vi "Refresh DiffIO Listbox.vi"(8 "Filters":sgl[](array[numeric]), 9 "Names":string[](array[string]), 10 "Setup":T1[](array[typedef]) caption="Differential I/O Setup" {"Skip Fire Index" max=7; "Angles"."Duration [s]" format="%#_3p"; "Frequency [Hz]" format="%#_3p"}, 11 "MulticolumnListbox in":refnum<vi>) -> ()   [LabVIEW 2016, in "DCM System Explorer.lvlib"]
uses:
  DCM System Explorer.lvlib
  <vilib>/Powertrain Controls/Device Drivers/DCM/Diff IO/RT/Setup.ctl
  <vilib>/Powertrain Controls/Device Drivers/DCM/Diff IO/FPGA/Mode.ctl
  <vilib>/Powertrain Controls/Device Drivers/DCM/Diff IO/RT/Angle Control.ctl
  <vilib>/Powertrain Controls/Device Drivers/DCM/Diff IO/RT/DCM - RT - Diff IO.lvlib
  <vilib>/Powertrain Controls/Device Drivers/DCM/Diff IO/FPGA/DCM - FPGA - Diff IO.lvlib
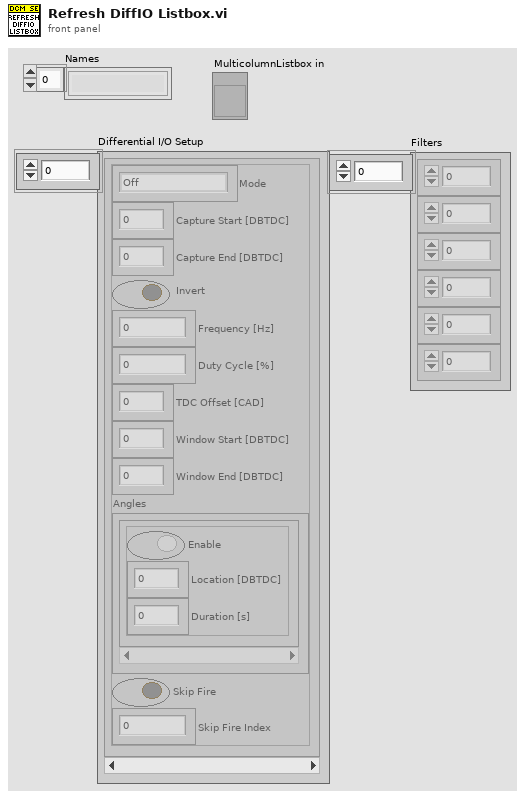
[diagram p1: front panel]
types:
  T1 = typedef "DCM - RT - Diff IO.lvlib/Setup.ctl" = cluster{"Mode":T2, "Capture Start [DBTDC]":sgl, "Capture End [DBTDC]":sgl, "Invert":bool, "Frequency [Hz]":sgl, "Duty Cycle [%]":sgl, "TDC Offset [CAD]":sgl, "Window Start [DBTDC]":sgl, "Window End [DBTDC]":sgl, "Angles":T3[], "Skip Fire":bool, "Skip Fire Index":u8}
  T2 = typedef "DCM - FPGA - Diff IO.lvlib/Mode.ctl" = enum8{"Off", "Input", "Pulse Width Modulation", "Engine Position Tracking", "Serial Out 1", "Serial Out 2", "EPTx Sync"}
  T3 = typedef "DCM - RT - Diff IO.lvlib/Angle Control.ctl" = cluster{"Enable":bool, "Location [DBTDC]":sgl, "Duration [s]":sgl}
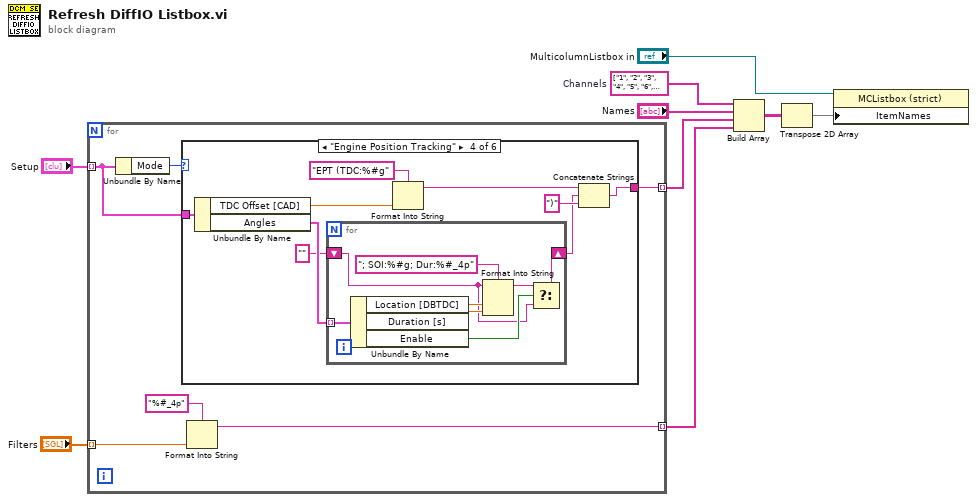
[diagram p0: block diagram]
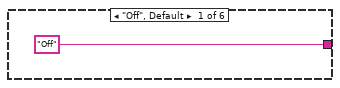
[diagram p2: hidden frame]
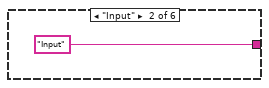
[diagram p3: hidden frame]
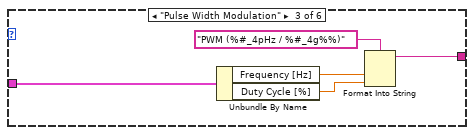
[diagram p4: hidden frame]
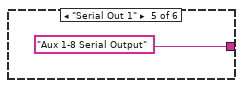
[diagram p5: hidden frame]
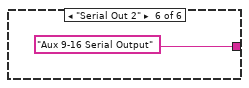
[diagram p6: hidden frame]
diagram:
  w8 = string[] ["1", "2", "3", "4", "5", "6", "7", "8"]  # Channels
  n1 = for {
    tunnel: "Setup" -> [w10] mode=indexing
    tunnel: [w11] -> w2 mode=indexing
    tunnel: "Filters" -> [w15] mode=indexing
    tunnel: [w13] -> w1 mode=indexing
    n2 = Unbundle By Name(w10) -> ("Mode"=w12:T2)
    n3 = case shown="\"Engine Position Tracking\"" w12 {
      tunnel: w10 -> [_ _ w22 w30 _ _]
      tunnel: ["Off" "Input" ("format string") w18 w26 "Aux 1-8 Serial Output" ("format string") "Aux 9-16 Serial Output" ("format string")] -> w11
      frame "Off", Default {
      }
      frame "Input" {
      }
      frame "Pulse Width Modulation" {
        n4 = Unbundle By Name(w22) -> ("Frequency [Hz]"=w20:sgl, "Duty Cycle [%]"=w19:sgl)
        n5 = Format Into String(format string="PWM (%#_4pHz / %#_4g%%)", w20, w19) -> (resulting string=w18:string)  [unwired: 2 in, 1 out]
      }
      frame "Engine Position Tracking" {
        n6 = Unbundle By Name(w30) -> ("TDC Offset [CAD]"=w29:sgl, "Angles"=w28:T3[])
        n7 = for {
          tunnel: w28 -> [w37] mode=indexing
          shift-right: [w33] -> w24
          shift-left: "" -> [w32]
          n8 = Unbundle By Name(w37) -> ("Location [DBTDC]"=w38:sgl, "Duration [s]"=w36:sgl, "Enable"=w35:bool)
          n9 = Format Into String(format string="; SOI:%#g; Dur:%#_4p", initial string=w32, w38, w36) -> (resulting string=w34:string)  [unwired: 1 in, 1 out]
          n10 = Select(t=w34, s=w35, f=w32) -> (s? t:f=w33:string)
        }
        n11 = Format Into String(format string="EPT (TDC:%#g", w29) -> (resulting string=w27:string)  [unwired: 2 in, 1 out]
        n12 = Concatenate Strings(w27, w24, ")" ("string")) -> (w26:string)
      }
      frame "Serial Out 1" {
      }
      frame "Serial Out 2" {
      }
    }
    n13 = Format Into String(format string="%#_4p", w15) -> (resulting string=w13:string)  [unwired: 2 in, 1 out]
  }
  n14 = Build Array(w8, "Names", w2, w1) -> (w9:string[][])
  n15 = Transpose 2D Array(2D array=w9) -> (transposed array=w7:string[][])
  n16 = property on="Property Node" class="MCListbox (strict)"(reference="MulticolumnListbox in", "ItemNames"=w7) -> ()  [unwired: 1 in, 2 out]
